vi "closest_angle.vi"(1 "b":dbl, 2 "a":dbl) -> (0 "dir":dbl)   [LabVIEW 2020]
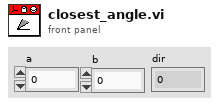
[diagram p1: front panel]
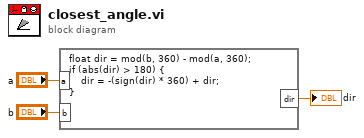
[diagram p0: block diagram]
diagram:
  n1 = formula code="float dir = mod(b, 360) - mod(a, 360);\nif (abs(dir) > 180) {\n    dir = -(sign(dir) * 360) + dir;\n}"("a"="a", "b"="b") -> ("dir"=→"dir":dbl)
